vi "UnloadSession.vi"(8 "error in (no error)":errorcluster, 11 "session id in":i32) -> (0 "error out":errorcluster, 2 "UnloadSession":bool, 3 "session id out":i32)   [LabVIEW 2018, in "libonnx_wrapper.lvlib"]
doc: "/**\n * @brief Выгрузить сессию из памяти (освободить веса модели)\n * \n * Эта функция освобождает память, занимаемую моделью (веса, вычислительный граф),\n * но сохраняет SessionID, путь к файлу и метаданные (имена входов/выходов, формы).\n * Позволяет временно освободить память и позже перезагрузить модель через ReloadSession.\n * \n * @param sessionId [IN] ID сессии для выгрузки\n * \n * @return int32: 0 при успешной выгрузке\n * @return int32: -1 если сессия не найдена\n * \n * @note Путь к модели сохраняется для возможности перезагрузки\n * @note SessionID остаётся валидным\n */\nint UnloadSession(int sessionId);"
uses:
  libonnx_wrapper.lvlib
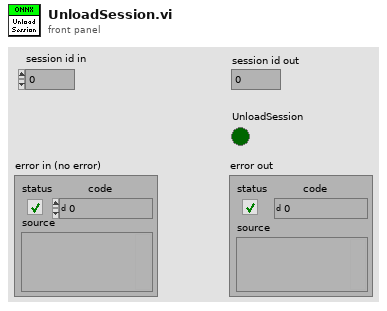
[diagram p1: front panel]
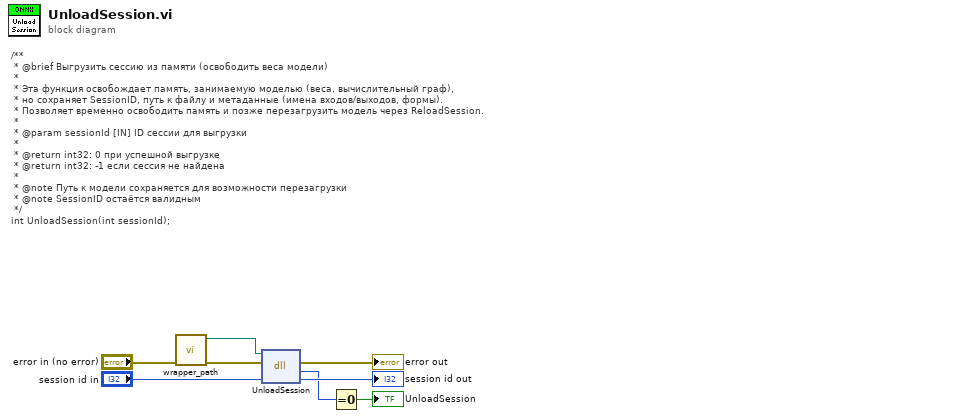
[diagram p0: block diagram]
diagram:
  # "/**\n * @brief Выгрузить сессию из памяти (освободить веса модели)\n * \n * Эта функция освобождает память, занимаемую моделью (веса, вычислительный граф),\n * но сохраняет SessionID, путь к файлу и метаданные (имена входов/выходов, формы).\n * Позволяет временно освободить память и позже перезагрузить модель через ReloadSession.\n * \n * @param sessionId [IN] ID сессии для выгрузки\n * \n * @return int32: 0 при успешной выгрузке\n * @return int32: -1 если сессия не найдена\n * \n * @note Путь к модели сохраняется для возможности перезагрузки\n * @note SessionID остаётся валидным\n */\nint UnloadSession(int sessionId);"
  n1 = call "wrapper_path.vi"("error in (no error)"="error in (no error)") -> ("error out"=w6:errorcluster, "wrapper path"=w5:path)  [unwired: 9 in]
  n2 = dll-call lib="home/ivan/LabVIEWData/ONNX/Test/libonnx_wrapper/unix64/libonnx_wrapper.so" fn="UnloadSession"(path in=w5, error in=w6, "sessionId"="session id in") -> (error out=→"error out":errorcluster, "UnloadSession"=w2:i32, "sessionId"=→"session id out":i32)  [unwired: 1 in, 1 out]
  n3 = Equal To 0?(x=w2) -> (x = 0?=→"UnloadSession":bool)
